vi "L1_RegisterInitialSetting.vi"(7 "REG ARRAy":u32[](array[numeric]), 8 "error in":errorcluster, 11 "connection ID in":refnum<k5>) -> (0 "error out":errorcluster, 3 "connection ID out":refnum<k5>)   [LabVIEW 2012]
panel:
  out "data out serial":string="empty_read_bufferwrittingempty_read_bufferwritting2"
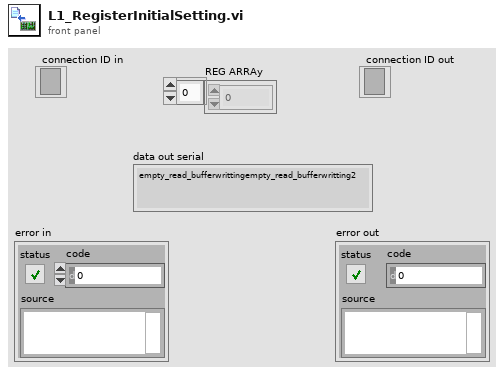
[diagram p1: front panel]
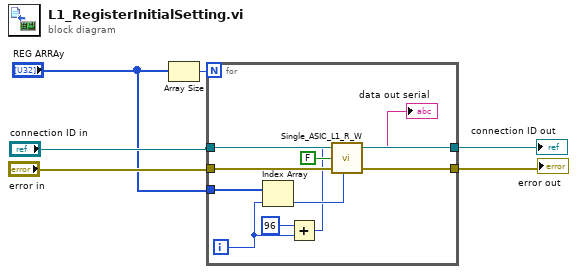
[diagram p0: block diagram]
diagram:
  n1 = Array Size(array="REG ARRAy") -> (size(s)=w6:i32)
  n2 = for {
    N: w6 -> [_]
    tunnel: "error in" -> [w17]
    tunnel: "REG ARRAy" -> [w16]
    tunnel: "connection ID in" -> [w15]
    tunnel: [w14] -> w4
    tunnel: [w13] -> w5
    i -> [w8]
    n3 = Index Array(array=w16, index=w8) -> (element=w12:u32)
    n4 = Add(x=96 ("y"), y=w8) -> (x+y=w10:i32)
    n5 = call "Single_ASIC_L1_R_W.vi"("connection ID"=w15, "Register or channel"=w10, "RD/#WR"=FALSE, "error in (no error)"=w17, "Data"=w12) -> ("data out serial"=→"data out serial":string, "connection ID out"=w14:refnum<k5>, "error out"=w13:errorcluster)  [unwired: 1 in, 1 out]
  }
  "error out" <- w5
  "connection ID out" <- w4
